vi "Right Justify.vi"(8 "error in":errorcluster, 10 "Position Coordinates":cluster{refnum<vi>, i32}[](array[cluster]), 11 "Splitter Reference":refnum<vi>) -> (0 "error out":errorcluster)   [LabVIEW 2013]
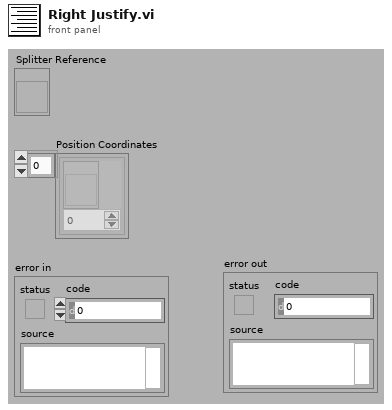
[diagram p1: front panel]
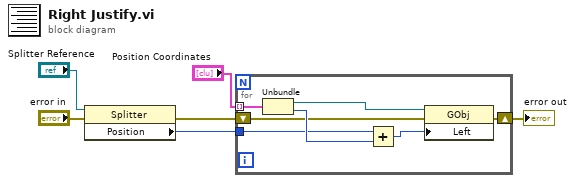
[diagram p0: block diagram]
diagram:
  n1 = property on="Property Node" class="Splitter"(reference="Splitter Reference", error in="error in") -> (error out=w3:errorcluster, "Position"=w1:i32)  [unwired: 1 out]
  n2 = for {
    tunnel: "Position Coordinates" -> [w12] mode=indexing
    shift-right: [w13] -> w5
    shift-left: w3 -> [w7]
    tunnel: w1 -> [w10]
    n3 = Unbundle(w12) -> (w8:refnum<vi>, w11:i32)
    n4 = Add(x=w10, y=w11) -> (x+y=w9:i32)
    n5 = property class="GObj"(reference=w8, error in=w7, "Left"=w9) -> (error out=w13:errorcluster)  [unwired: 1 out]
  }
  "error out" <- w5
